vi "Volatus Post-Build Action.vi"(5 "Files Generated by Build":path[](array[path]), 6 "Top Level/Always Included VIs":path[](array[path]), 7 "Destination Path":path, 8 "error in (no error)":errorcluster, 9 "Target Name":string, 10 "Build Specification Name":string, 11 "Project Path":path) -> (0 "error out":errorcluster)   [LabVIEW 2020, in "VolatusBuild.lvlib"]
uses:
  VolatusBuild.lvlib
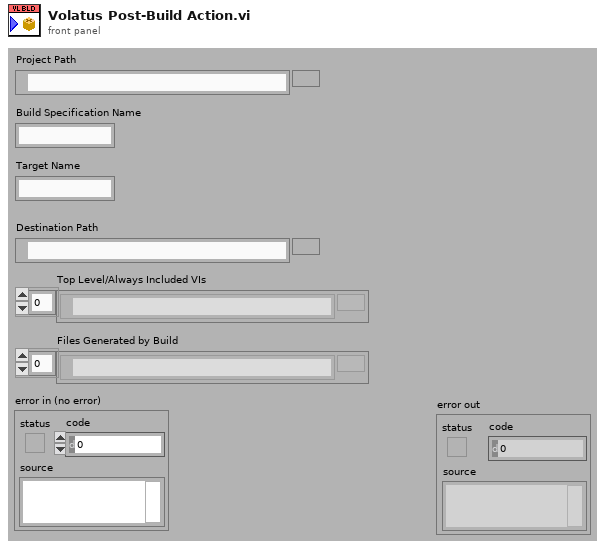
[diagram p1: front panel]
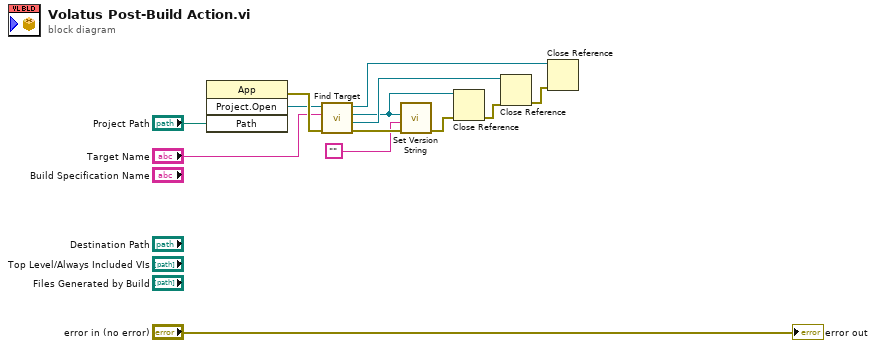
[diagram p0: block diagram]
diagram:
  n1 = invoke class="App" method="Project.Open"("Path"="Project Path") -> (error out=w12:errorcluster, "Project:Open"=w11:refnum<vi>)  [unwired: 3 in, 2 out]
  n2 = call "Find Target.vi"("error in (no error)"=w12, "Target"="Target Name", "Project in"=w11) -> ("error out"=w2:errorcluster, "Target"=w9:refnum<vi>, "TargetAppContext"=w6:refnum<vi>, "Project"=w7:refnum<vi>)  [unwired: 5 in]
  n3 = call "Set Version String.vi"("error in (no error)"=w2, "Version String"="", "App"=w6) -> ("error out"=w5:errorcluster)  [unwired: 8 in]
  n4 = Close Reference(reference=w6, error in (no error)=w5) -> (error out=w10:errorcluster)
  n5 = Close Reference(reference=w9, error in (no error)=w10) -> (error out=w8:errorcluster)
  n6 = Close Reference(reference=w7, error in (no error)=w8) -> ()  [unwired: 1 out]
  "error out" <- "error in (no error)"
